vi "Read Attributes.vi"(11 "Test Window Launched Msg":refnum<class "Test Window Launched Msg.lvclass">) -> (2 "Payload":T1)   [LabVIEW 2017, in "Test.lvlib" / "Test Window Launched Msg.lvclass"]
uses:
  Test Window Launched Msg.lvclass
  Test Window Launched Msg.lvclass/Test Window Launched Msg.ctl
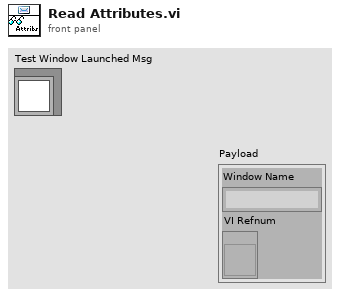
[diagram p1: front panel]
types:
  T1 = cluster{"Window Name":string, "VI Refnum":refnum<vi>}
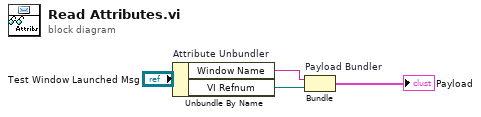
[diagram p0: block diagram]
diagram:
  n1 = Unbundle By Name "Attribute Unbundler"("Test Window Launched Msg") -> ("Window Name"=w2:string, "VI Refnum"=w1:refnum<vi>)
  n2 = Bundle "Payload Bundler"("Window Name"=w2, "VI Refnum"=w1) -> (→"Payload":T1)  [unwired: 1 in]
